vi "CRC.vi"(11 "命令字符串":string) -> (3 "校验字符串":string)   [LabVIEW 2017]
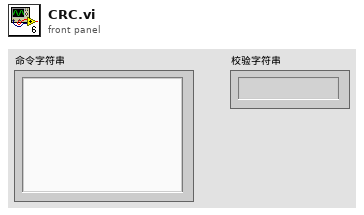
[diagram p1: front panel]
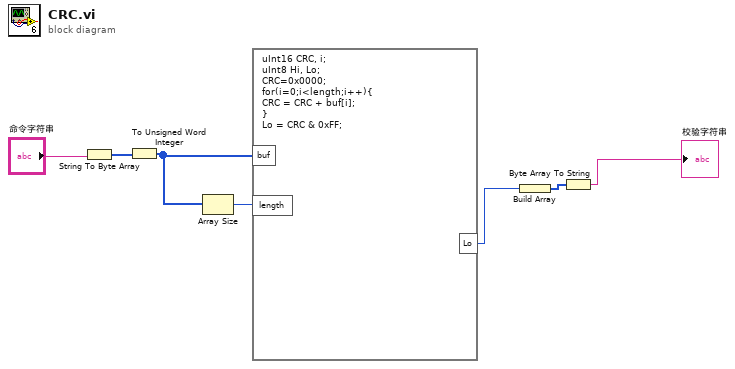
[diagram p0: block diagram]
diagram:
  n1 = String To Byte Array(string="命令字符串") -> (unsigned byte array=w6:u8[])
  n2 = To Unsigned Word Integer(number=w6) -> (unsigned 16bit integer=w4:u16[])
  n3 = Array Size(array=w4) -> (size(s)=w5:i32)
  n4 = formula code="uInt16 CRC, i;\nuInt8 Hi, Lo;\nCRC=0x0000;\nfor(i=0;i<length;i++){\nCRC = CRC + buf[i];\n}\nLo = CRC & 0xFF;"("length"=w5, "buf"=w4) -> ("Lo"=w3:u8)
  n5 = Build Array(w3) -> (w2:u8[])
  n6 = Byte Array To String(unsigned byte array=w2) -> (string=→"校验字符串":string)
